vi "DeleteAudioValidationServices.vi"   [LabVIEW 2021]
types:
  T1 = enum32{"Invalid", "Standard", "Closed", "Hidden", "Minimized", "Maximized"}
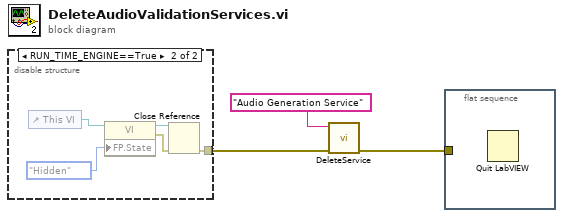
[diagram p0: block diagram]
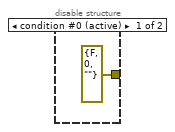
[diagram p2: hidden frame]
diagram:
  n1 = disable-structure shown="RUN_TIME_ENGINE==True" {
    disable-tunnel: [errorcluster {"status"=FALSE, "code"=0, "source"=""} ("error in (no error)") w5] -> w1
    frame condition #0 (active) {
    }
    frame condition #1 {
      n2 = control-ref of="This VI"() -> (w8:refnum<vi>)
      n3 = property class="VI"(reference=w8, "FP.State"=T1."Hidden" ("Front Panel Window:State")) -> (reference out=w7:refnum<vi>, error out=w6:errorcluster)  [unwired: 1 in]
      n4 = Close Reference(reference=w7, error in (no error)=w6) -> (error out=w5:errorcluster)
    }
  }
  n5 = call "DeleteService.vi"("error in (no error)"=w1, "service name"="Audio Generation Service") -> ("error out"=w2:errorcluster)  [unwired: 9 in]
  n6 = flat-sequence {
    tunnel: w2 -> [_]
    frame #0 {
      n7 = Quit LabVIEW() -> ()  [unwired: 1 in]
    }
  }
